vi "Tflop.vi"(3 "Pulse":bool) -> (0 "Qnot":bool, 1 "Q":bool)   [LabVIEW 2015]
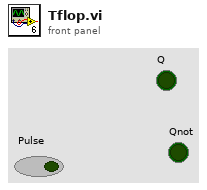
[diagram p1: front panel]
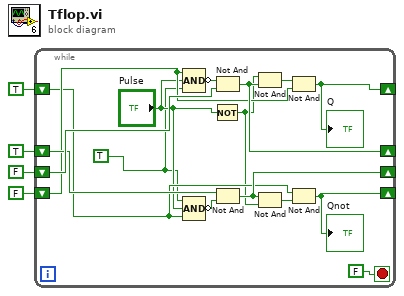
[diagram p0: block diagram]
diagram:
  n1 = while {
    shift-right: [w7] -> _
    shift-left: FALSE -> [w11]
    shift-right: [w16] -> _
    shift-left: TRUE -> [w18]
    shift-right: [w8] -> _
    shift-left: TRUE -> [w10]
    shift-right: [w17] -> _
    shift-left: FALSE -> [w19]
    stop <- FALSE stop-if-true
    w5 = TRUE
    n2 = Compound Arithmetic op=AND(w11, "Pulse", w5) -> (invert w14:bool)
    n3 = Compound Arithmetic op=AND(w5, "Pulse", w10) -> (invert w15:bool)
    n4 = Not(x="Pulse") -> (.not. x?=w9:bool)
    n5 = Not And(1:w19, 2:w14) -> (0:w16:bool)
    n6 = Not And(1:w15, 2:w18) -> (0:w17:bool)
    n7 = Not And(1:w16, 2:w9) -> (0:w13:bool)
    n8 = Not And(1:w9, 2:w17) -> (0:w12:bool)
    n9 = Not And(1:w11, 2:w13) -> (0:w8:bool)
    "Q" <- w8
    n10 = Not And(1:w12, 2:w10) -> (0:w7:bool)
    "Qnot" <- w7
  }
